vi "Interpreted Data.vi"(3 "Input":dbl[](array[numeric]), 4 "Interpreted Data FGV Selector":T1, 5 "Action":T2) -> (0 "Output":dbl[](array[numeric]))   [LabVIEW 2013]
uses:
  Functional Globals/Action.ctl
  Interpreted Data FGV Selector.ctl
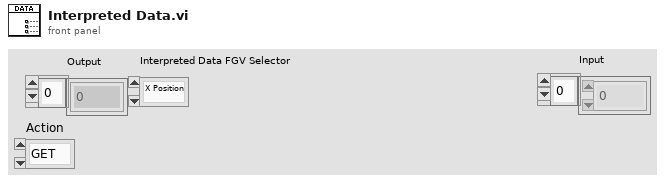
[diagram p1: front panel]
types:
  T1 = typedef "Interpreted Data FGV Selector.ctl" = enum16{"X Position", "Y Position", "Z Position", "Force", "Signal Strength"}
  T2 = typedef "Action.ctl" = enum16{"GET", "PUT", "DELETE"}
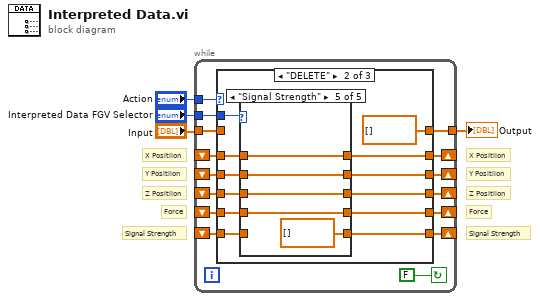
[diagram p0: block diagram]
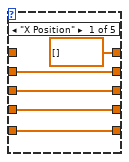
[diagram p7: hidden frame]
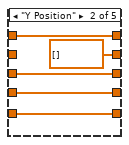
[diagram p8: hidden frame]
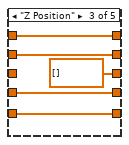
[diagram p9: hidden frame]
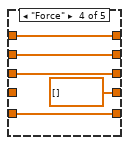
[diagram p10: hidden frame]
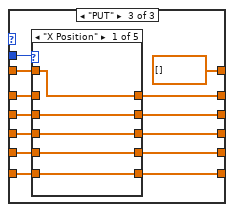
[diagram p11: hidden frame]
diagram:
  # "Signal Strength"
  # "Signal Strength"
  # "Force"
  # "Force"
  # "Z Positiion"
  # "Z Positiion"
  # "Y Positiion"
  # "Y Positiion"
  # "X Positiion"
  # "X Positiion"
  n1 = while {
    tunnel: [w16] -> w4
    tunnel: "Input" -> [w17]
    tunnel: "Action" -> [w19]
    tunnel: "Interpreted Data FGV Selector" -> [w18]
    shift-right: [w13] -> _
    shift-left: _ -> [w15]
    shift-right: [w12] -> _
    shift-left: _ -> [w14]
    shift-right: [w11] -> _
    shift-left: _ -> [w10]
    shift-right: [w9] -> _
    shift-left: _ -> [w8]
    shift-right: [w7] -> _
    shift-left: _ -> [w6]
    stop <- FALSE continue-if-true
    n2 = case shown="\"DELETE\"" w19 {
      tunnel: w18 -> [w31 w68 w106]
      tunnel: w17 -> [_ _ w95]
      tunnel: [w20 dbl[] [] ("Input") dbl[] [] ("Input")] -> w16
      tunnel: w15 -> [w30 w67 w105]
      tunnel: w14 -> [w29 w66 w104]
      tunnel: [w28 w65 w103] -> w13
      tunnel: [w27 w64 w102] -> w12
      tunnel: [w26 w63 w101] -> w11
      tunnel: w10 -> [w25 w62 w100]
      tunnel: [w24 w61 w99] -> w9
      tunnel: w8 -> [w23 w60 w98]
      tunnel: [w22 w59 w97] -> w7
      tunnel: w6 -> [w21 w58 w96]
      frame "GET" {
        n3 = case shown="\"X Position\"" w31 {
          tunnel: w30 -> [w32 w41 w46 w51 w56]
          tunnel: w29 -> [w36 w37 w45 w50 w55]
          tunnel: [w32 w41 w46 w51 w56] -> w28
          tunnel: [w36 w37 w45 w50 w55] -> w27
          tunnel: [w35 w40 w42 w49 w54] -> w26
          tunnel: w25 -> [w35 w40 w42 w49 w54]
          tunnel: [w34 w39 w44 w47 w53] -> w24
          tunnel: w23 -> [w34 w39 w44 w47 w53]
          tunnel: [w33 w38 w43 w48 w52] -> w22
          tunnel: w21 -> [w33 w38 w43 w48 w52]
          tunnel: [w32 w37 w42 w47 w52] -> w20
          frame "X Position" {
          }
          frame "Y Position" {
          }
          frame "Z Position" {
          }
          frame "Force" {
          }
          frame "Signal Strength" {
          }
        }
      }
      frame "DELETE" {
        n4 = case shown="\"Signal Strength\"" w68 {
          tunnel: w67 -> [_ w78 w83 w88 w93]
          tunnel: w66 -> [w73 _ w82 w87 w92]
          tunnel: [dbl[] [] ("Input") w78 w83 w88 w93] -> w65
          tunnel: [w73 dbl[] [] ("Input") w82 w87 w92] -> w64
          tunnel: [w72 w77 dbl[] [] ("Input") w86 w91] -> w63
          tunnel: w62 -> [w72 w77 _ w86 w91]
          tunnel: [w71 w76 w81 dbl[] [] ("Input") w90] -> w61
          tunnel: w60 -> [w71 w76 w81 _ w90]
          tunnel: [w70 w75 w80 w85 dbl[] [] ("Input")] -> w59
          tunnel: w58 -> [w70 w75 w80 w85 _]
          frame "X Position" {
          }
          frame "Y Position" {
          }
          frame "Z Position" {
          }
          frame "Force" {
          }
          frame "Signal Strength" {
          }
        }
      }
      frame "PUT" {
        n5 = case shown="\"X Position\"" w106 {
          tunnel: w105 -> [_ w116 w121 w126 w131]
          tunnel: w104 -> [w111 _ w120 w125 w130]
          tunnel: [w107 w116 w121 w126 w131] -> w103
          tunnel: [w111 w112 w120 w125 w130] -> w102
          tunnel: [w110 w115 w117 w124 w129] -> w101
          tunnel: w100 -> [w110 w115 _ w124 w129]
          tunnel: [w109 w114 w119 w122 w128] -> w99
          tunnel: w98 -> [w109 w114 w119 _ w128]
          tunnel: [w108 w113 w118 w123 w127] -> w97
          tunnel: w96 -> [w108 w113 w118 w123 _]
          tunnel: w95 -> [w107 w112 w117 w122 w127]
          frame "X Position" {
          }
          frame "Y Position" {
          }
          frame "Z Position" {
          }
          frame "Force" {
          }
          frame "Signal Strength" {
          }
        }
      }
    }
  }
  "Output" <- w4
